vi "Untitled 1.vi"() -> ()   [LabVIEW 2011]
panel:
  out "x-y":u32
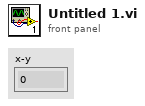
[diagram p1: front panel]
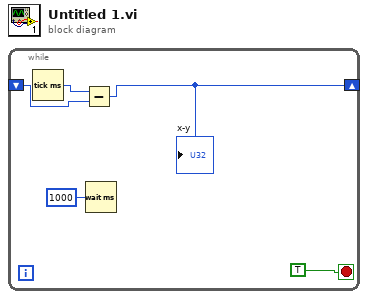
[diagram p0: block diagram]
diagram:
  n1 = while {
    shift-right: [w3] -> _
    shift-left: _ -> [w2]
    stop <- TRUE stop-if-true
    n2 = Tick Count (ms)() -> (millisecond timer value=w4:u32)
    n3 = Subtract(x=w4, y=w2) -> (x-y=w3:u32)
    "x-y" <- w3
    n4 = Wait (ms)(milliseconds to wait=u32 1000) -> ()  [unwired: 1 out]
  }
